vi "2_Boolean_Adder(Inference).vi"() -> ()   [LabVIEW 2020]
uses:
  <vilib>/Ngene/Deep Learning Toolkit/Toolkit/NN_Network/Controls/NN_Save_Before_Destroy_Options.ctl
  <vilib>/Ngene/Deep Learning Toolkit/Toolkit/NN_Network/API/NN_Set_Input/1D/NN_Set_Input(1D_SGL_idx).vi
  <vilib>/Ngene/Deep Learning Toolkit/Toolkit/Deep_Learning_Toolkit_by_Ngene.lvlib
panel:
  out "C(Ground Truth)":u8=11
  out "C(Predicted)":u8=11
  in  "?":bool
  in  "A":u8=7
  in  "B":u8=4
  in  "Weight File":path=path "D:/Ngene/GitHub/deepltk_examples/1_Simple_Examples/13_Boolean_Adder_Logistic_Regresion/working/Adder 8bit/Adder 8bit_weights_23_08_03__19_09_51.bin"
  in  "CFG File":path=path "D:/Ngene/GitHub/deepltk_examples/1_Simple_Examples/13_Boolean_Adder_Logistic_Regresion/working/Adder 8bit/Adder 8bit_net_cfg_23_08_03__19_09_51.cfg"
  # "Overview: Demonstrates the usage of DeepLTK for loading the model pretrained for modeling 8-bit Boolean adder.\nRequirements: DeepLTK - Deep Learning Toolkit for LabVIEW (https://www.ngene.co/deep-learning-toolkit-for-labview)\n\nInstructions:\n1. Provide Network Configuration File Path and Weight File Path generated from \"1_Boolean_Adder_Logistic_Regression(Train).vi\".\n2. Run the VI.\n3. Provide ader's inputs at A and B controls.\n4. Observe the prediction of the network at C(Predicted) indicator.\n5. Press the Stop button to stop the VI.\n\nMore Examples:  https://github.com/ngenehub/deepltk_examples"
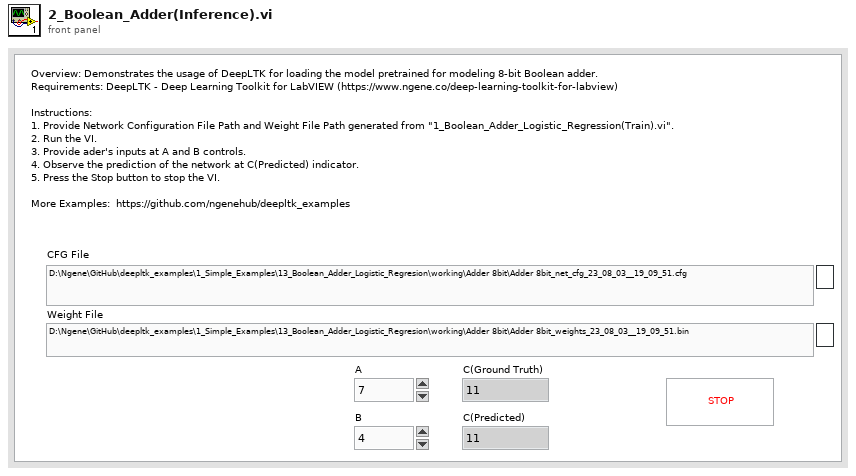
[diagram p1: front panel]
types:
  T1 = typedef "Deep_Learning_Toolkit_by_Ngene.lvlib/NN_Save_Before_Destroy_Options.ctl" = cluster{"CFG?":bool, "Weights?":bool, "Render?":bool}
  T2 = typedef "Deep_Learning_Toolkit_by_Ngene.lvlib/NN_Config_Params.ctl" = cluster{"Name":string, "mBatch":i32, "NN_Train_Params":T3, "LR_Decay_Policy":T6, "Labels":string[], "Loss":T8}
  T3 = typedef "Deep_Learning_Toolkit_by_Ngene.lvlib/NN_Train_Params.ctl" = cluster{"Optimizer":T4, "Beta_1":sgl, "Beta_2":sgl, "Weight Decay(L1)":sgl, "Weight Decay(L2)":sgl, "Data_Sampling":T5}
  T4 = typedef "Deep_Learning_Toolkit_by_Ngene.lvlib/NN_Train_Optimizer.ctl" = enum16{"SGD", "Adam", "Adagrad", "Adadelta", "RMSProp", "Nesterov"}
  T5 = typedef "Deep_Learning_Toolkit_by_Ngene.lvlib/NN_Train_Data_Sampling.ctl" = enum16{"Random", "Sequential"}
  T6 = typedef "Deep_Learning_Toolkit_by_Ngene.lvlib/NN_LR_Policy_Cfg.ctl" = cluster{"Policy_Type":T7, "LR0":dbl, "k":sgl, "WarmUp_Policy":enum16{"Step", "Ramp"}, "WarmUp_Iter":i32, "WarmUp_Ratio":sgl}
  T7 = typedef "Deep_Learning_Toolkit_by_Ngene.lvlib/NN_LR_Policy_Type.ctl" = enum16{"Manual", "Step", "Exp", "1/t"}
  T8 = typedef "Deep_Learning_Toolkit_by_Ngene.lvlib/NN_Loss_Config_Params.ctl" = cluster{"Loss_Type":T9, "Loss_Conf_Params":variant}
  T9 = typedef "Deep_Learning_Toolkit_by_Ngene.lvlib/NN_Loss_Type.ctl" = enum16{"None", "MSE", "CrossEntropy", "YOLO_v2", "YOLO_v4"}
  T10 = typedef "Deep_Learning_Toolkit_by_Ngene.lvlib/NN_Layer_Config_Params.ctl" = cluster{"Layer_Type":T11, "Layer_Conf_Params":variant, "Input Layers":string[]}
  T11 = typedef "Deep_Learning_Toolkit_by_Ngene.lvlib/NN_Layer_Type.ctl" = enum16{"Input1D", "Input3D", "Conv1D", "Conv2D", "Conv2D_Adv", "MaxPool", "AvgPool", "UpSample", "DropOut3D", "ShortCut", "Concat", "SoftMax3D", "FC", "DropOut", "Softmax", "Flatten", "YOLO_v2", "YOLO_v4", "Activation", "BatchNormalization", "Unsupported"}
  T12 = typedef "Deep_Learning_Toolkit_by_Ngene.lvlib/NN.ctl" = cluster{"Name":string, "No of Layers":i32, "mBatch":i32, "Layers":T13[], "Dimty":T14, "Dims_In":T15, "Dims_Out":T15, "Working_Dir":path, "Train?":bool, "Train_Params":T3, "LR_Update_Policy":T6, "Session Data":T16, "Ground_truth":T17, "NNg_hdls":T18, "NN_Device":T19, "GPU Id":i32, "Labels":string[], "Receptive Field":T20[], "Loss_Type":T9, "Loss_Cfg_Prms":variant, "NNG_WS":T21}
  T13 = typedef "Deep_Learning_Toolkit_by_Ngene.lvlib/NN_Layer_ref.ctl" = refnum<data-value>
  T14 = typedef "Deep_Learning_Toolkit_by_Ngene.lvlib/NN_In_Out_Dim-ty.ctl" = enum8{"In1D_Out1D", "In3D_Out1D", "In3D_Out3D", "In3D_OutBBox"}
  T15 = typedef "Deep_Learning_Toolkit_by_Ngene.lvlib/NN_Dims(C,H,W).ctl" = cluster{"C":i32, "H":i32, "W":i32}
  T16 = typedef "Deep_Learning_Toolkit_by_Ngene.lvlib/NN_Train_Session_Data.ctl" = cluster{"Epochs":sgl, "Tot_Iter":i32, "LR":sgl, "LR_iter":i32}
  T17 = typedef "Deep_Learning_Toolkit_by_Ngene.lvlib/NN_Ground_truth.ctl" = cluster{"Y":variant}
  T18 = typedef "Deep_Learning_Toolkit_by_Ngene.lvlib/nng_cuda_handles.ctl" = cluster{"cudnn":u64, "cublas":u64, "stream":u64, "curand":u64}
  T19 = typedef "Deep_Learning_Toolkit_by_Ngene.lvlib/NN_Device.ctl" = enum16{"CPU", "GPU"}
  T20 = typedef "Deep_Learning_Toolkit_by_Ngene.lvlib/NN_Dims(V,H).ctl" = cluster{"V":i32, "H":i32}
  T21 = typedef "Deep_Learning_Toolkit_by_Ngene.lvlib/NNG_WS.ctl" = cluster{"NNG_WS_Mem":T22, "Max_WS_Size":i64}
  T22 = typedef "Deep_Learning_Toolkit_by_Ngene.lvlib/NNg_WS_Mem_DVR.ctl" = refnum<data-value>
  T23 = typedef "Deep_Learning_Toolkit_by_Ngene.lvlib/NN_Layer.ctl" = cluster{"Name":string, "Layer_Data":variant, "Layer_Type":T11, "Dims_In":T15, "Layers_In":variant, "Dims_Out":T15, "Layers_Out":variant, "Metrics":T24, "GPU_Data":variant, "mBatch":i32, "NN_Device":T19, "NNg_hdls":T18, "Train?":bool, "Dimty":T25, "RecptField":T26}
  T24 = typedef "Deep_Learning_Toolkit_by_Ngene.lvlib/NN_Layer_Metrics.ctl" = cluster{"Data":dbl, "Params":dbl, "Ops":dbl}
  T25 = typedef "Deep_Learning_Toolkit_by_Ngene.lvlib/NN_Layer_Dimty.ctl" = enum16{"1D", "3D"}
  T26 = typedef "Deep_Learning_Toolkit_by_Ngene.lvlib/NN_Layer_RF_State.ctl" = cluster{"Dims":T20, "J":T20}
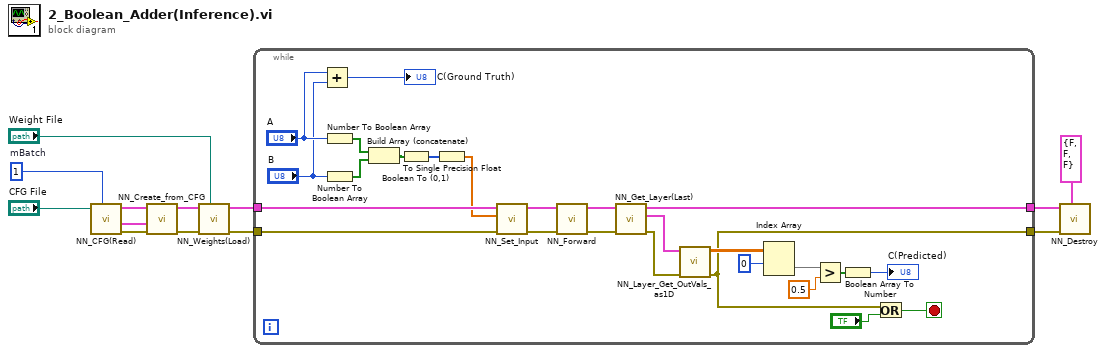
[diagram p0: block diagram]
diagram:
  w13 = 1  # mBatch
  n1 = call <vilib>:"NN_CFG(Read).vi"("mBatch"=w13, "CFG file path"="CFG File") -> ("error out"=w10:errorcluster, "Net_Cfg"=w11:T2, "Layer_Cfg"=w2:T10[])  [unwired: 7 in]
  n2 = call <vilib>:"NN_Create_from_CFG.vi"("error in (no error)"=w10, "Net_Cfg"=w11, "Layer_Cfg"=w2) -> ("error out"=w8:errorcluster, "NN out"=w9:T12)  [unwired: 7 in]
  n3 = call <vilib>:"NN_Weights(Load).vi"("Weight File Path"="Weight File", "error in (no error)"=w8, "NN in"=w9) -> ("error out"=w5:errorcluster, "NN out"=w6:T12)  [unwired: 7 in]
  n4 = while {
    tunnel: w6 -> [w39]
    tunnel: w5 -> [w38]
    tunnel: [w29] -> w4
    tunnel: [w23] -> w3
    stop <- w24 stop-if-true
    n5 = Add(x="A", y="B") -> (x+y=→"C(Ground Truth)":u8)
    n6 = Number To Boolean Array(number="A") -> (Boolean array=w37:bool[])
    n7 = Number To Boolean Array(number="B") -> (Boolean array=w14:bool[])
    n8 = Build Array (concatenate)(w37, w14) -> (w15:bool[])
    n9 = Boolean To (0,1)(Boolean=w15) -> (0, 1=w36:i16[])
    n10 = To Single Precision Float(number=w36) -> (single precision float=w22:sgl[])
    n11 = call-poly <vilib>:"NN_Set_Input.vi"("error in (no error)"=w38, "Data_In(1D_SGL)"=w22, "NN In"=w39) -> ("error out"=w34:errorcluster, "NN Out"=w35:T12)  [unwired: 7 in]
    n12 = call <vilib>:"NN_Forward.vi"("error in (no error)"=w34, "NN in"=w35) -> ("error out"=w32:errorcluster, "NN out"=w33:T12)  [unwired: 6 in, 2 out]
    n13 = call <vilib>:"NN_Get_Layer(Last).vi"("error in (no error)"=w32, "NN in"=w33) -> ("error out"=w30:errorcluster, "Last_Layer"=w31:T23, "NN out"=w29:T12)  [unwired: 6 in, 1 out]
    n14 = call <vilib>:"NN_Layer_Get_OutVals_as1D.vi"("error in (no error)"=w30, "Layer"=w31) -> ("error out"=w23:errorcluster, "Out(as1D)"=w28:sgl[][])  [unwired: 8 in]
    n15 = Index Array(array=w28, index (row)=0) -> (element=w26:sgl[])  [unwired: 1 in]
    n16 = Greater?(x=w26, y=sgl 0.5) -> (0:w18:bool[])
    n17 = Boolean Array To Number(Boolean array=w18) -> (number=→"C(Predicted)":u8)
    n18 = Or(x=w23, y="?") -> (x .or. y?=w24:bool)
  }
  n19 = call <vilib>:"NN_Destroy.vi"("Save (T, T, T)"=T1 {"CFG?"=FALSE, "Weights?"=FALSE, "Render?"=FALSE}, "error in (no error)"=w3, "NN in"=w4) -> ()  [unwired: 7 in, 2 out]
